vi "U32-Array-to-U8-Array.vi"(11 "U32 [] in":u32[](array[numeric]) format="%.0x") -> (3 "U8 [] out":u8[](array[numeric]) format="%.0x")   [LabVIEW 2018]
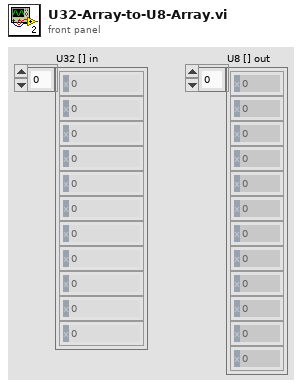
[diagram p1: front panel]
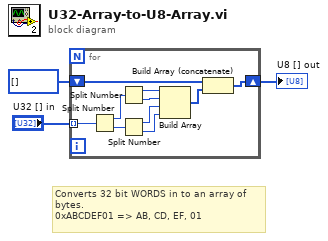
[diagram p0: block diagram]
diagram:
  # "Converts 32 bit WORDS in to an array of\nbytes.\n0xABCDEF01 => AB, CD, EF, 01"
  n1 = for {
    tunnel: "U32 [] in" -> [w13] mode=indexing
    shift-right: [w5] -> w3
    shift-left: u8[] [] -> [w4]
    n2 = Split Number(x=w13) -> (hi(x)=w12:u16, lo(x)=w11:u16)
    n3 = Split Number(x=w12) -> (hi(x)=w10:u8, lo(x)=w9:u8)
    n4 = Split Number(x=w11) -> (hi(x)=w8:u8, lo(x)=w7:u8)
    n5 = Build Array(w10, w9, w8, w7) -> (w6:u8[])
    n6 = Build Array (concatenate)(w4, w6) -> (w5:u8[])
  }
  "U8 [] out" <- w3
